vi "EvaluateLabeledExpression.vi"(6 "AllowMissingLabels":bool, 8 "error in (no error)":errorcluster, 10 "Expression":string, 11 "Labels":cluster{"Label":string, "Value":string}[](array[cluster])) -> (0 "error out":errorcluster, 1 "Log":T1, 2 "Result":bool)   [LabVIEW 2021, in "Expressions.lvlib"]
uses:
  Expressions.lvlib
  <vilib>/gmath/NI_Gmath.lvlib
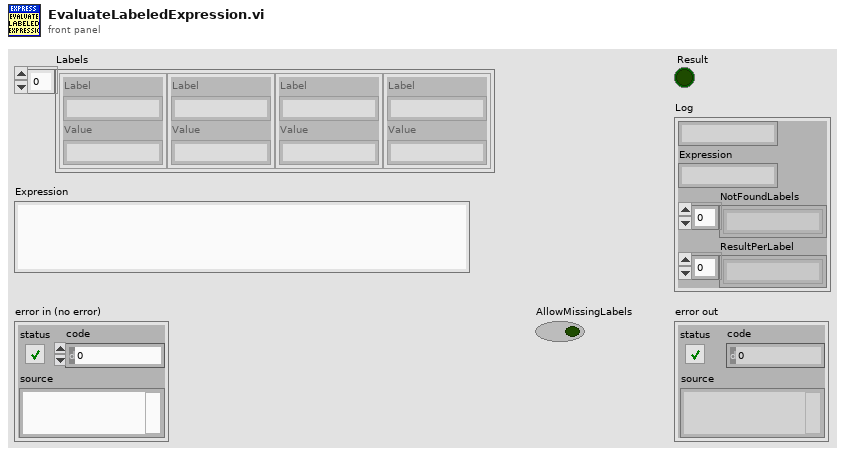
[diagram p1: front panel]
types:
  T1 = cluster{string, "Expression":string, "NotFoundLabels":string[], "ResultPerLabel":string[]}
  T2 = cluster{string, "Expression":string, string[], string[]}
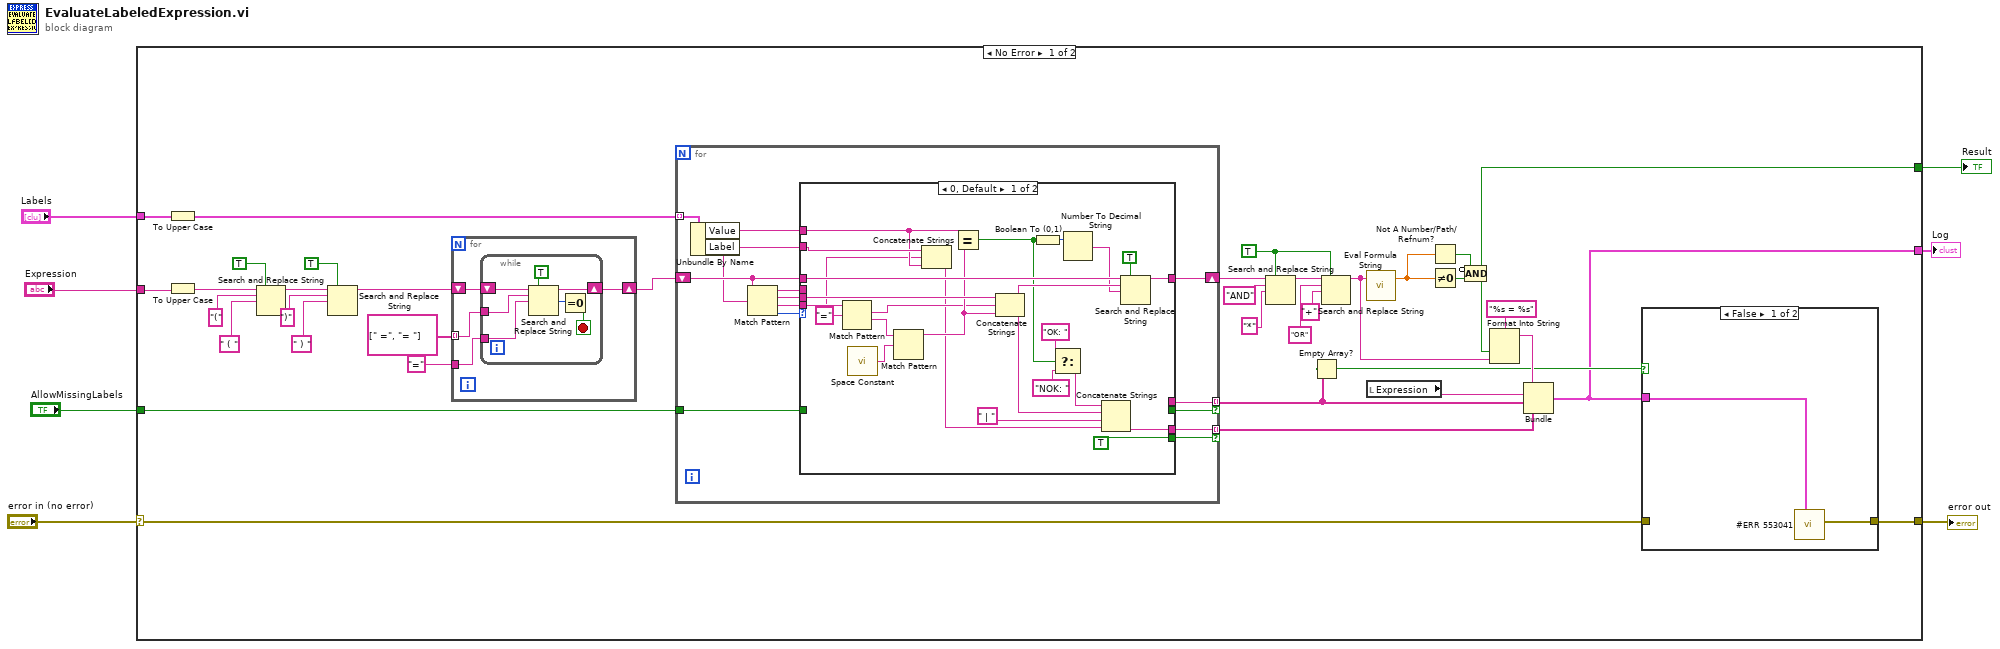
[diagram p0: block diagram]
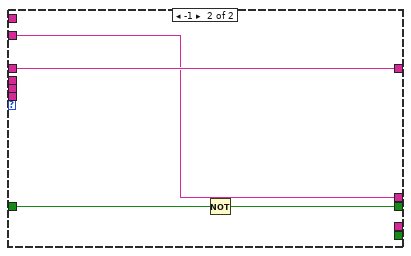
[diagram p3: hidden frame]
diagram:
  n1 = case shown="No Error" "error in (no error)" {
    selector: "error in (no error)" -> [w17 w100]
    tunnel: "Labels" -> [w44 _]
    tunnel: "Expression" -> [w42 _]
    tunnel: [w16 w100] -> w4
    tunnel: [w9 _] -> w3
    tunnel: "AllowMissingLabels" -> [w15 _]
    tunnel: [w8 _] -> w1
    frame No Error {
      w35 = TRUE ("replace all? (F)")
      n2 = To Upper Case(1:w44) -> (0:w43:cluster{"Label":string, "Value":string}[])
      n3 = To Upper Case(1:w42) -> (0:w32:string)
      n4 = Search and Replace String(replace all?=TRUE ("replace all? (F)"), input string=w32, search string="(", replace string=" ( " ("search string")) -> (result string=w27:string)  [unwired: 4 in, 3 out]
      n5 = Search and Replace String(replace all?=TRUE ("replace all? (F)"), input string=w27, search string=")", replace string=" ) " ("search string")) -> (result string=w26:string)  [unwired: 4 in, 3 out]
      n6 = for {
        shift-right: [w50] -> w23
        shift-left: w26 -> [w51]
        tunnel: string[] [" =", "= "] -> [w49] mode=indexing
        tunnel: "=" ("search string") -> [w48]
        n7 = while {
          shift-right: [w57] -> w50
          shift-left: w51 -> [w58]
          tunnel: w49 -> [w55]
          tunnel: w48 -> [w54]
          stop <- w53 stop-if-true
          n8 = Search and Replace String(replace all?=TRUE, input string=w58, search string=w55, replace string=w54) -> (result string=w57:string, number of replacements=w52:i32)  [unwired: 4 in, 2 out]
          n9 = Equal To 0?(x=w52) -> (x = 0?=w53:bool)
        }
      }
      n10 = for {
        tunnel: w43 -> [w72] mode=indexing
        shift-right: [w65] -> w41
        shift-left: w23 -> [w67]
        tunnel: [w64] -> w14 mode=indexing if=w63
        tunnel: [w62] -> w21 mode=indexing if=w61
        tunnel: w15 -> [w59]
        n11 = Unbundle By Name(w72) -> ("Value"=w68:string, "Label"=w60:string)
        n12 = Match Pattern(string=w67, regular expression=w60) -> (before substring=w69:string, match substring=w66:string, after substring=w70:string, offset past match=w71:i32)  [unwired: 1 in]
        n13 = case shown="0, Default" w71 {
          tunnel: w70 -> [w95 _]
          tunnel: w69 -> [_ _]
          tunnel: w68 -> [w78 _]
          tunnel: w67 -> [w92 w99]
          tunnel: w66 -> [w91 _]
          tunnel: [w88 w99] -> w65
          tunnel: [_ w98] -> w64
          tunnel: [_ w96] -> w63
          tunnel: [w83 _] -> w62
          tunnel: [TRUE _] -> w61
          tunnel: w60 -> [w79 w98]
          tunnel: w59 -> [_ w97]
          frame 0, Default {
            w77 = "=" ("regular expression")
            n14 = Match Pattern(string=w95, regular expression=w77) -> (match substring=w81:string, after substring=w94:string)  [unwired: 1 in, 2 out]
            n15 = call <vilib>:"Space Constant.vi"() -> ("String"=w93:string)
            n16 = Match Pattern(string=w94, regular expression=w93) -> (before substring=w82:string)  [unwired: 1 in, 3 out]
            n17 = Concatenate Strings(w79, w77, w78) -> (w80:string)
            n18 = Equal?(x=w78, y=w82) -> (x = y?=w76:bool)
            n19 = Concatenate Strings(w91, w81, w82) -> (w86:string)
            n20 = Boolean To (0,1)(Boolean=w76) -> (0, 1=w89:i16)
            n21 = Select(t="OK: ", s=w76, f="NOK: ") -> (s? t:f=w73:string)
            n22 = Number To Decimal String(number=w89) -> (decimal integer string=w85:string)  [unwired: 1 in]
            n23 = Concatenate Strings(w73, w86, " | ", w80) -> (w83:string)
            n24 = Search and Replace String(replace all?=TRUE ("replace all? (F)"), input string=w92, search string=w86, replace string=w85) -> (result string=w88:string)  [unwired: 4 in, 3 out]
          }
          frame -1 {
            n25 = Not(x=w97) -> (.not. x?=w96:bool)
          }
        }
      }
      n26 = Search and Replace String(replace all?=w35, input string=w41, search string="AND", replace string="*" ("replace string (\"\")")) -> (result string=w40:string)  [unwired: 4 in, 3 out]
      n27 = Empty Array?(array=w14) -> (empty?=w13:bool)
      n28 = Search and Replace String(replace all?=w35, input string=w40, search string="OR", replace string="+" ("search string")) -> (result string=w19:string)  [unwired: 4 in, 3 out]
      n29 = call <vilib>:"Eval Formula String.vi"("formula"=w19) -> ("y value"=w12:dbl)  [unwired: 1 in, 1 out]
      n30 = local read "Expression"() -> (w22:string)
      n31 = Not A Number/Path/Refnum?(number/path/refnum=w12) -> (NaN/Path/Refnum?=w10:bool)
      n32 = Not Equal To 0?(x=w12) -> (x != 0?=w11:bool)
      n33 = Compound Arithmetic op=AND(invert w10, w11) -> (w9:bool)
      n34 = Format Into String(format string="%s = %s", w9, w19) -> (resulting string=w18:string)  [unwired: 2 in, 1 out]
      n35 = Bundle(w18, "Expression"=w22, w14, w21) -> (w8:T2)  [unwired: 1 in]
      n36 = case shown="False" w13 {
        tunnel: [w46 w47] -> w16
        tunnel: w8 -> [w45 _]
        tunnel: w17 -> [_ w47]
        frame False {
          n37 = call "#ERR 553041"("Data"=w45) -> ("error out"=w46:errorcluster)  [unwired: 10 in]
        }
        frame True {
        }
      }
    }
    frame Error {
    }
  }
  "error out" <- w4
  "Result" <- w3
  "Log" <- w1
